vi "Get Minion ID.vi"() -> (3 "minion id":string)   [LabVIEW 2017]
uses:
  <vilib>/Utility/sysdir.llb/System Directory Type.ctl
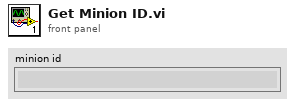
[diagram p1: front panel]
types:
  T1 = typedef "System Directory Type.ctl" = i32
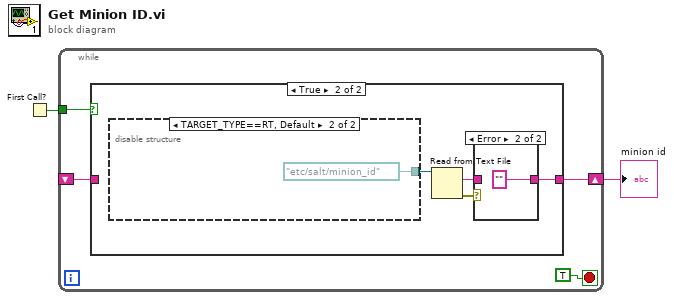
[diagram p0: block diagram]
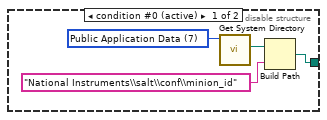
[diagram p4: hidden frame]
diagram:
  n1 = First Call?() -> (First Call?: T/F=w1:bool)
  n2 = while {
    tunnel: w1 -> [w5]
    shift-right: [w6] -> w2
    shift-left: _ -> [w3]
    stop <- TRUE stop-if-true
    n3 = case shown="True" w5 {
      tunnel: [w7 w8] -> w6
      tunnel: w3 -> [w7 _]
      frame False {
      }
      frame True {
        n4 = disable-structure shown="TARGET_TYPE==RT, Default" {
          disable-tunnel: [w14 path "/etc/salt/minion_id" ("file (use dialog)")] -> w11
          frame condition #0 (active) {
            w17 = T1 7 items=["User Home"=0, "User Desktop"=1, "User Documents"=2, "User Application Data"=3, "User Preferences"=4, "User Temporary"=5, "Public Documents"=6, "Public Application Data"=7, "Public Preferences"=8, "Public Cache"=13, "System Core Libraries"=9, "System Installed Libraries"=10, "Application Files"=11, "Boot Volume Root"=12] ("system directory type")
            n5 = call <vilib>:"Get System Directory.vi"("system directory type"=w17) -> ("system directory"=w15:path)  [unwired: 10 in]
            n6 = Build Path(base path=w15, name or relative path="National Instruments\\salt\\conf\\minion_id") -> (appended path=w14:path)
          }
          frame condition #1 {
          }
        }
        n7 = Read from Text File(file (use dialog)=w11) -> (text=w9:string, error out=w10:errorcluster)  [unwired: 3 in, 2 out]
        n8 = case shown="Error" w10 {
          tunnel: w9 -> [w12 _]
          tunnel: [w12 ""] -> w8
          frame No Error {
          }
          frame Error {
          }
        }
      }
    }
  }
  "minion id" <- w2
